vi "Cash Karp General.vi"(4 "X":string[](array[string])=["x1", "x2"], 5 "result":dbl[][](array[numeric]) format="%.2f", 6 "time":string="t", 7 "table":i32[][][](array[numeric]), 8 "zero":dbl[](array[numeric])=[0.0, 0.0, 0.0, 0.0, 0.0, 0.0] format="%.4f", 9 "yn":dbl[](array[numeric]) format="%.2f", 10 "xn":dbl format="%.2f", 11 "h":dbl=1.0 format="%.2f") -> (2 "yn2":dbl[](array[numeric]) format="%.2f", 3 "yn1":dbl[](array[numeric]) format="%.2f")   [LabVIEW 2014, in "NI_Gmath.lvlib"]
uses:
  NI_Gmath.lvlib
  Real Dot Product.vi
  NI_AALBase.lvlib
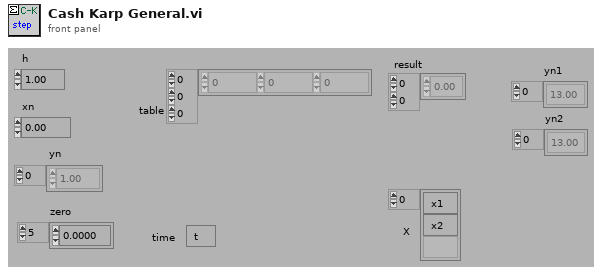
[diagram p1: front panel]
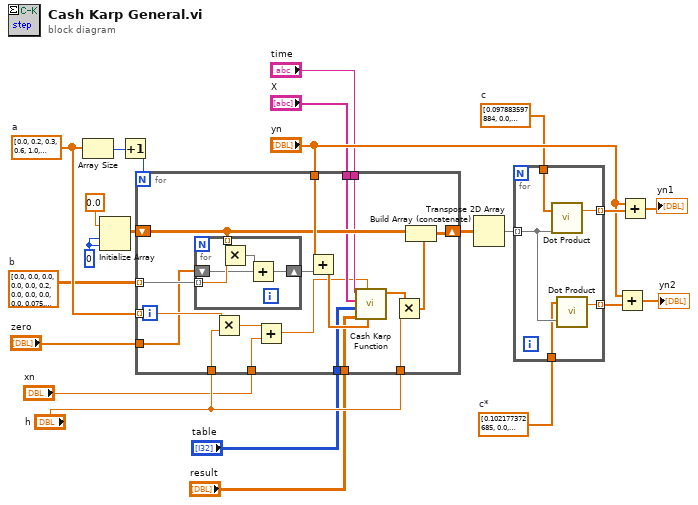
[diagram p0: block diagram]
diagram:
  w6 = dbl[] [0.102177372685, 0.0, 0.383907903439, 0.244592737269, 0.019321986607, 0.25]  # c*
  w7 = dbl[] [0.097883597884, 0.0, 0.402576489533, 0.210437710438, 0.0, 0.289102202146]  # c
  w8 = dbl[][] [[0.0, 0.0, 0.0, 0.0, 0.0], [0.2, 0.0, 0.0, 0.0, 0.0], [0.075, 0.225, 0.0, 0.0, 0.0], [0.3, -0.9, 1.2, 0.0, 0.0], [-0.2037, 2.5, -2.592592592593, 1.296296296296, 0.0], [0.029495804398, 0.341796875, 0.041594328704, 0.400345413773, 0.061767578125]]  # b
  w9 = dbl[] [0.0, 0.2, 0.3, 0.6, 1.0, 0.875]  # a
  w12 = 0
  n1 = Array Size(array=w9) -> (size(s)=w19:i32)
  n2 = Initialize Array(0.0, w12, w12) -> (w23:dbl[][])
  n3 = Increment(x=w19) -> (x+1=w18:i32)
  n4 = for {
    N: w18 -> [_]
    shift-right: [w37] -> w17
    shift-left: w23 -> [w35]
    tunnel: "h" -> [w42]
    tunnel: w9 -> [w40] mode=indexing
    tunnel: "h" -> [w41]
    tunnel: w8 -> [w34] mode=indexing
    tunnel: "xn" -> [w39]
    tunnel: "yn" -> [w36]
    tunnel: "zero" -> [w29]
    tunnel: "time" -> [w28]
    tunnel: "X" -> [w27]
    tunnel: "table" -> [w26]
    tunnel: "result" -> [w25]
    n5 = for {
      shift-right: [w43] -> w33
      shift-left: w29 -> [w45]
      tunnel: w35 -> [w47] mode=indexing
      tunnel: w34 -> [w46] mode=indexing
      n6 = Multiply(x=w47, y=w46) -> (x*y=w44:dbl[])
      n7 = Add(x=w44, y=w45) -> (x+y=w43:dbl[])
    }
    n8 = Multiply(x=w40, y=w41) -> (x*y=w38:dbl)
    n9 = Add(x=w38, y=w39) -> (x+y=w24:dbl)
    n10 = Add(x=w36, y=w33) -> (x+y=w30:dbl[])
    n11 = call "Cash Karp Function.vi"(6:"X"=w30, 7:"time"=w24, "result"=w25, "table"=w26, 10:"X"=w27, 11:"time"=w28) -> ("F(X,time)"=w32:dbl[])  [unwired: 5 in]
    n12 = Multiply(x=w32, y=w42) -> (x*y=w31:dbl[])
    n13 = Build Array (concatenate)(w35, w31) -> (w37:dbl[][])
  }
  n14 = Transpose 2D Array(2D array=w17) -> (transposed array=w10:dbl[][])
  n15 = for {
    tunnel: [w52] -> w11 mode=indexing
    tunnel: w10 -> [w51] mode=indexing
    tunnel: [w50] -> w20 mode=indexing
    tunnel: w7 -> [w49]
    tunnel: w6 -> [w48]
    n16 = call-poly "Dot Product.vi"("Y Vector"=w51, "X Vector"=w49) -> ("X * Y"=w50:dbl)  [unwired: 1 out]
    n17 = call-poly "Dot Product.vi"("Y Vector"=w51, "X Vector"=w48) -> ("X * Y"=w52:dbl)  [unwired: 1 out]
  }
  n18 = Add(x="yn", y=w11) -> (x+y=→"yn2":dbl[])
  n19 = Add(x="yn", y=w20) -> (x+y=→"yn1":dbl[])
